vi "WhatForebrainPerception.vi"(3 "What?Midbrain":cluster{"T":dbl, "Range":dbl, "Bearing":dbl}[](array[cluster])) -> (1 "What?Midbrain 2":cluster{"T":dbl, "Range":dbl, "Bearing":dbl}[](array[cluster]))   [LabVIEW 2012]
doc: "This SubVI takes clean Whatsense data from the Midbrain and layers perception onto it to be passed to the THINK processes in the Forebrain\n\nT=time\nRange\nBearing"
panel:
  # "This SubVI adds \nperception onto the\nWhere data comming\nfrom the Midbrain"
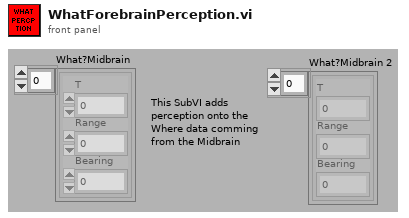
[diagram p1: front panel]
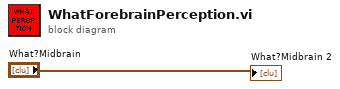
[diagram p0: block diagram]
diagram:
  "What?Midbrain 2" <- "What?Midbrain"
